vi "Open and Configure FPGA.vi"(8 "error in":errorcluster, 11 "resource name":T2) -> (0 "error out":errorcluster, 3 "FPGA VI Reference Out":T1)   [LabVIEW 2018, in "RT-FPGA Interface API.lvlib"]
uses:
  RT-FPGA Interface API.lvlib
  <vilib>/userdefined/High Color/nirio_resource_hc.ctl
  FPGA ref.ctl
  <vilib>/FPGAPlugInAG/cRIO-9118/niLvFpga_Open_cRIO-9118.vi
  <vilib>/rvi/interface/common/dynamic/niFpgaDynamicAddResources.vi
  <vilib>/FPGAPlugInAG/Dynamic/niLvFpga_Reset_Dynamic.vi
  <vilib>/FPGAPlugInAG/Dynamic/niLvFpga_Run_Dynamic.vi
  <vilib>/Utility/error.llb/Error Cluster From Error Code.vi
  <vilib>/rvi/errors/niLvFpgaAdjustHostInterfaceError.vi
  <vilib>/rvi/interface/nirviOpenFPGA/nirviOpenFPGA.xnode
  FPGA Bitfiles/SistemadeControl_FPGATarget_FPGAmain_BFayZ0A1nnk.lvbitx
  <vilib>/rvi/interface/nirviMethod/nirviMethod.xnode
  <vilib>/rvi/interface/nirviReadWriteControl/nirviReadWriteControl.xnode
  NiFpgaLv.dll
  <vilib>/rvi/interface/Simulation/niFpgaSimulationCallBeginRW.vi
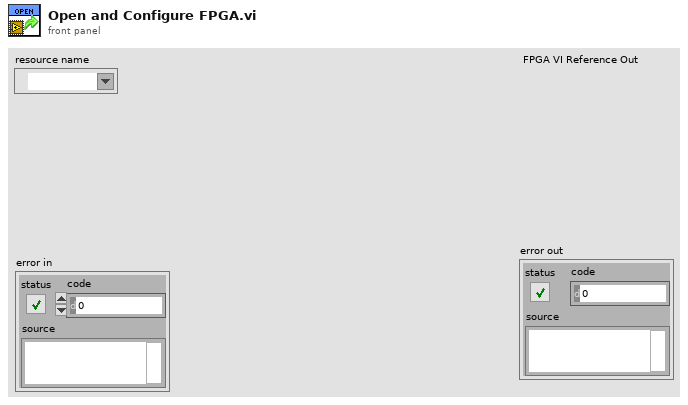
[diagram p1: front panel]
types:
  T1 = typedef "RT-FPGA Interface API.lvlib/FPGA ref.ctl" = refnum<k20>
  T2 = typedef "nirio_resource_hc.ctl" = tag
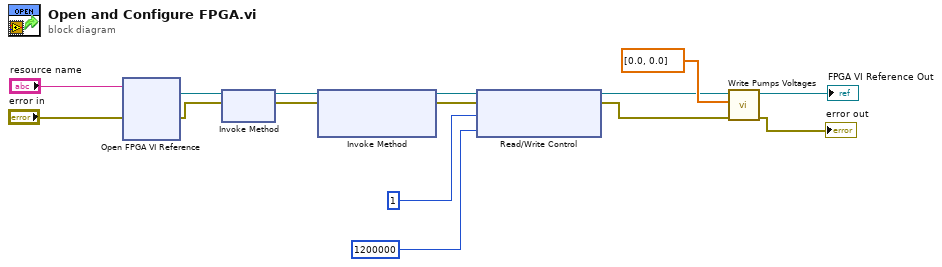
[diagram p0: block diagram]
diagram:
  n1 = xnode "Open FPGA VI Reference"("error in"="error in", "resource name"="resource name") -> ("FPGA VI Reference Out"=w15:refnum<k20>, "error out"=w13:errorcluster)
  n2 = xnode "Invoke Method"("FPGA VI Reference In"=w15, "error in"=w13) -> ("FPGA VI Reference Out"=w14:refnum<k20>, "error out"=w12:errorcluster)
  n3 = xnode "Invoke Method"("FPGA VI Reference In"=w14, "error in"=w12) -> ("FPGA VI Reference Out"=w9:refnum<k20>, "error out"=w8:errorcluster)  [unwired: 1 in]
  n4 = xnode "Read/Write Control"("FPGA VI Reference In"=w9, "error in"=w8, "Temporização FPGA"=u32 1, "Safe wait"=u32 1200000) -> ("FPGA VI Reference Out"=w4:refnum<k20>, "error out"=w2:errorcluster)
  n5 = call "Write Pumps Voltages.vi"("error in (no error)"=w2, "Pumps Voltages"=dbl[] [0.0, 0.0], "FPGA VI Reference In"=w4) -> ("error out"=→"error out":errorcluster, "FPGA VI Reference Out"=→"FPGA VI Reference Out":refnum<k20>)  [unwired: 7 in]
